vi "Truncate_Excessive_Strings.vi"(2 "Max String Length":i32=1500, 3 "String":string) -> (1 "Truncated String":string)   [LabVIEW 2022 SP3]
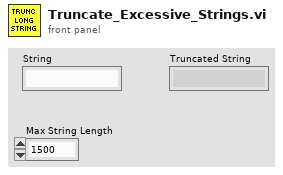
[diagram p1: front panel]
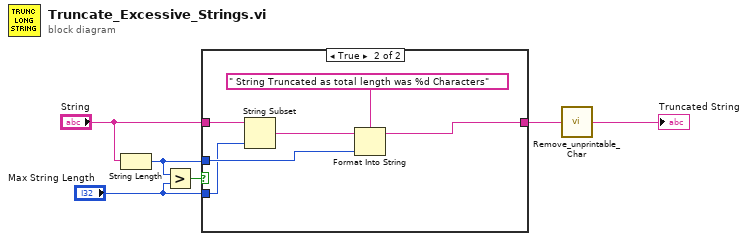
[diagram p0: block diagram]
diagram:
  n1 = String Length(string="String") -> (length=w5:i32)
  n2 = Greater?(x=w5, y="Max String Length") -> (0:w3:bool)
  n3 = case shown="True" w3 {
    tunnel: [w7 w8] -> w2
    tunnel: "String" -> [w7 w13]
    tunnel: "Max String Length" -> [_ w9]
    tunnel: w5 -> [_ w12]
    frame False {
    }
    frame True {
      n4 = String Subset(string=w13, length (rest)=w9) -> (substring=w11:string)  [unwired: 1 out]
      n5 = Format Into String(format string=" String Truncated as total length was %d Characters", initial string=w11, w12) -> (resulting string=w8:string)  [unwired: 1 in, 1 out]
    }
  }
  n6 = call "Remove_unprintable_Char.vi"("Input String"=w2) -> ("Output String"=→"Truncated String":string)
